vi "624WPI_DriverStationStart Communication.vi"(8 "error out":errorcluster, 11 "occurrence":refnum<k4>) -> ()   [LabVIEW 2013]
doc: "Starts the communication loop between the CompactRIO device and the driver station. This VI also initializes the host computer, joystick, and driver station data caches, as well as the system watchdog on the CompactRIO device.\n\nThis software is licensed. Open the labview\\readme\\WPI Robotics Library Open Source License.txt file for more information."
uses:
  <vilib>/Rock Robotics/WPI/DriverStation/WPI_DriverStationStatusErrorCache.ctl
  <vilib>/Rock Robotics/SystemInterfaces/NetworkCommunication/NetComm_UsageReport_ResourceType.ctl
  <vilib>/Rock Robotics/WPI/DriverStation/WPI_DriverStationLaptopDataCacheOp.ctl
  <vilib>/Rock Robotics/WPI/Joystick/WPI_JoystickCacheOp.ctl
  <vilib>/Rock Robotics/WPI/DriverStation/WPI_DriverStationCommDataCacheOp.ctl
  <vilib>/Rock Robotics/WPI/DriverStation/Enhanced IO/WPI_Enhanced IORaw Output Operation Mode.ctl
  <vilib>/Rock Robotics/WPI/DriverStation/WPI_DriverStationStatusDataCache.ctl
  <vilib>/Rock Robotics/WPI/Joystick/WPI_JoystickDeviceDataRaw.ctl
  <vilib>/Rock Robotics/WPI/DriverStation/WPI_DriverStationAllianceInfoCacheOp.ctl
  <vilib>/Rock Robotics/WPI/AnalogModule/WPI_AnalogModuleGetAverageVoltage.vi
  <vilib>/Utility/error.llb/Clear Errors.vi
panel:
  out "STOPCOMM":bool
  # "This VI start the communication loop and cache data for LabVIEW."
  # "VI MODIFIED - To use analog 8 (battery voltage) for speedier measurement\nin robot code, for correcting pressure readouts, etc."
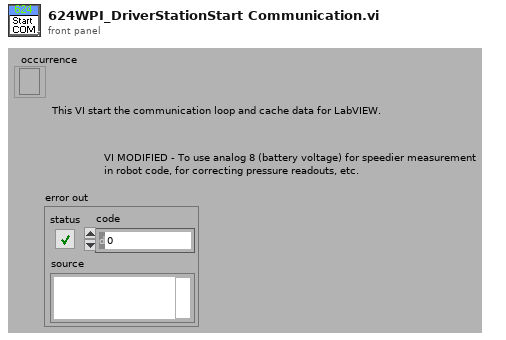
[diagram p1: front panel]
types:
  T1 = typedef "NetComm_UsageReport_ResourceType.ctl" = enum8{"Controller", "Module", "Language", "CANPlugin", "Accelerometer", "ADXL345", "AnalogChannel", "AnalogTrigger", "AnalogTriggerOutput", "CANJaguar", "Compressor", "Counter", "Dashboard", "DigitalInput", "DigitalOutput", "DriverStationCIO", "DriverStationEIO", "DriverStationLCD", "Encoder", "GearTooth", "Gyro", "I2C", "Framework", "Jaguar", "Joystick", "Kinect", "KinectStick", "PIDController", "Preferences", "PWM", "Relay", "RobotDrive", "SerialPort", "Servo", "Solenoid", "SPI", "Task", "Ultrasonic", "Victor", "Button", "Command", "AxisCamera", "PCVideoServer", "SmartDashboard", "Talon", "HiTechnicColorSensor", "HiTechnicAccel", "HiTechnicCompass", "SRF08"}
  T2 = typedef "WPI_DriverStationStatusErrorCache.ctl" = enum16{"Get", "Set"}
  T3 = typedef "WPI_DriverStationCommDataCacheOp.ctl" = enum16{"Get", "Set", "Init"}
  T4 = typedef "WPI_JoystickCacheOp.ctl" = enum16{"Set", "Init", "Get"}
  T5 = typedef "WPI_DriverStationLaptopDataCacheOp.ctl" = enum16{"Get", "Set", "Init"}
  T6 = typedef "WPI_JoystickDeviceDataRaw.ctl" = cluster{"axis 1":i8, "axis 2":i8, "axis 3":i8, "axis 4":i8, "axis 5":i8, "axis 6":i8, "Buttons":u16}
  T7 = typedef "WPI_DriverStationStatusDataCache.ctl" = enum16{"Get", "Set Digital Output", "Set High Priority Data", "Set Low Priority Data"}
  T8 = typedef "WPI_Enhanced IORaw Output Operation Mode.ctl" = enum16{"Get", "Set LEDs", "Set Digital Outputs", "Set Analog Outputs", "Set Digital Configuration", "Set PWMs", "Set All", "Invalidate", "Send Extended Bit", "Clear Extended Bit"}
  T9 = typedef "WPI_DriverStationAllianceInfoCacheOp.ctl" = enum16{"Get", "Set", "Init"}
  T10 = typedef "WPI_Enhanced IODataIn.ctl" = cluster{"api_version":u8, "fw_version":u8, "analog":cluster{"analog[0]":i16, "analog[1]":i16, "analog[2]":i16, "analog[3]":i16, "analog[4]":i16, "analog[5]":i16, "analog[6]":i16, "analog[7]":i16}, "digital":u16, "accel":cluster{"accel[0]":i16, "accel[1]":i16, "accel[2]":i16}, "quad":cluster{"quad[0]":i16, "quad[1]":i16}, "buttons":u8, "capsense slider":u8, "capsense prox":u8}
  T11 = typedef "WPI_Enhanced IODataOut.ctl" = cluster{"digital":u16, "digital_oe":u16, "digital_pe":u16, "pwm1_compare1":u16, "pwm1_compare2":u16, "pwm2_compare1":u16, "pwm2_compare2":u16, "pwm1_period":u16, "pwm2_period":u16, "dac1":u8, "dac2":u8, "leds":u8, "enables":u8, "dig_out":u8}
  T12 = typedef "WPI_DriverStationCommPacketData.ctl" = cluster{"packetIndex":u16, "control":u8, "dsDigitalIn":u8, "teamID":u16, "dsIDAlliance":u8, "dsIDPosition":u8, "J0 Axis 1":i8, "J0 Axis 2":i8, "J0 Axis 3":i8, "J0 Axis 4":i8, "J0 Axis 5":i8, "J0 Axis 6":i8, "J0 Buttons":u16, "J1 Axis 1":i8, "J1 Axis 2":i8, "J1 Axis 3":i8, "J1 Axis 4":i8, "J1 Axis 5":i8, "J1 Axis 6":i8, "J1 Buttons":u16, "J2 Axis 1":i8, "J2 Axis 2":i8, "J2 Axis 3":i8, "J2 Axis 4":i8, "J2 Axis 5":i8, "J2 Axis 6":i8, "J2 Buttons":u16, "J3 Axis 1":i8, "J3 Axis 2":i8, "J3 Axis 3":i8, "J3 Axis 4":i8, "J3 Axis 5":i8, "J3 Axis 6":i8, "J3 Buttons":u16, "analog 1":u16, "analog 2":u16, "analog 3":u16, "analog 4":u16, "cRIO checksum":u64, "FPGA checksum1":u64, "FPGA checksum2":u64, "vMonth1":u8, "vMonth2":u8, "vDay1":u8, "vDay2":u8, "vYear1":u8, "vYear2":u8, "vRev1":u8, "vRev2":u8}
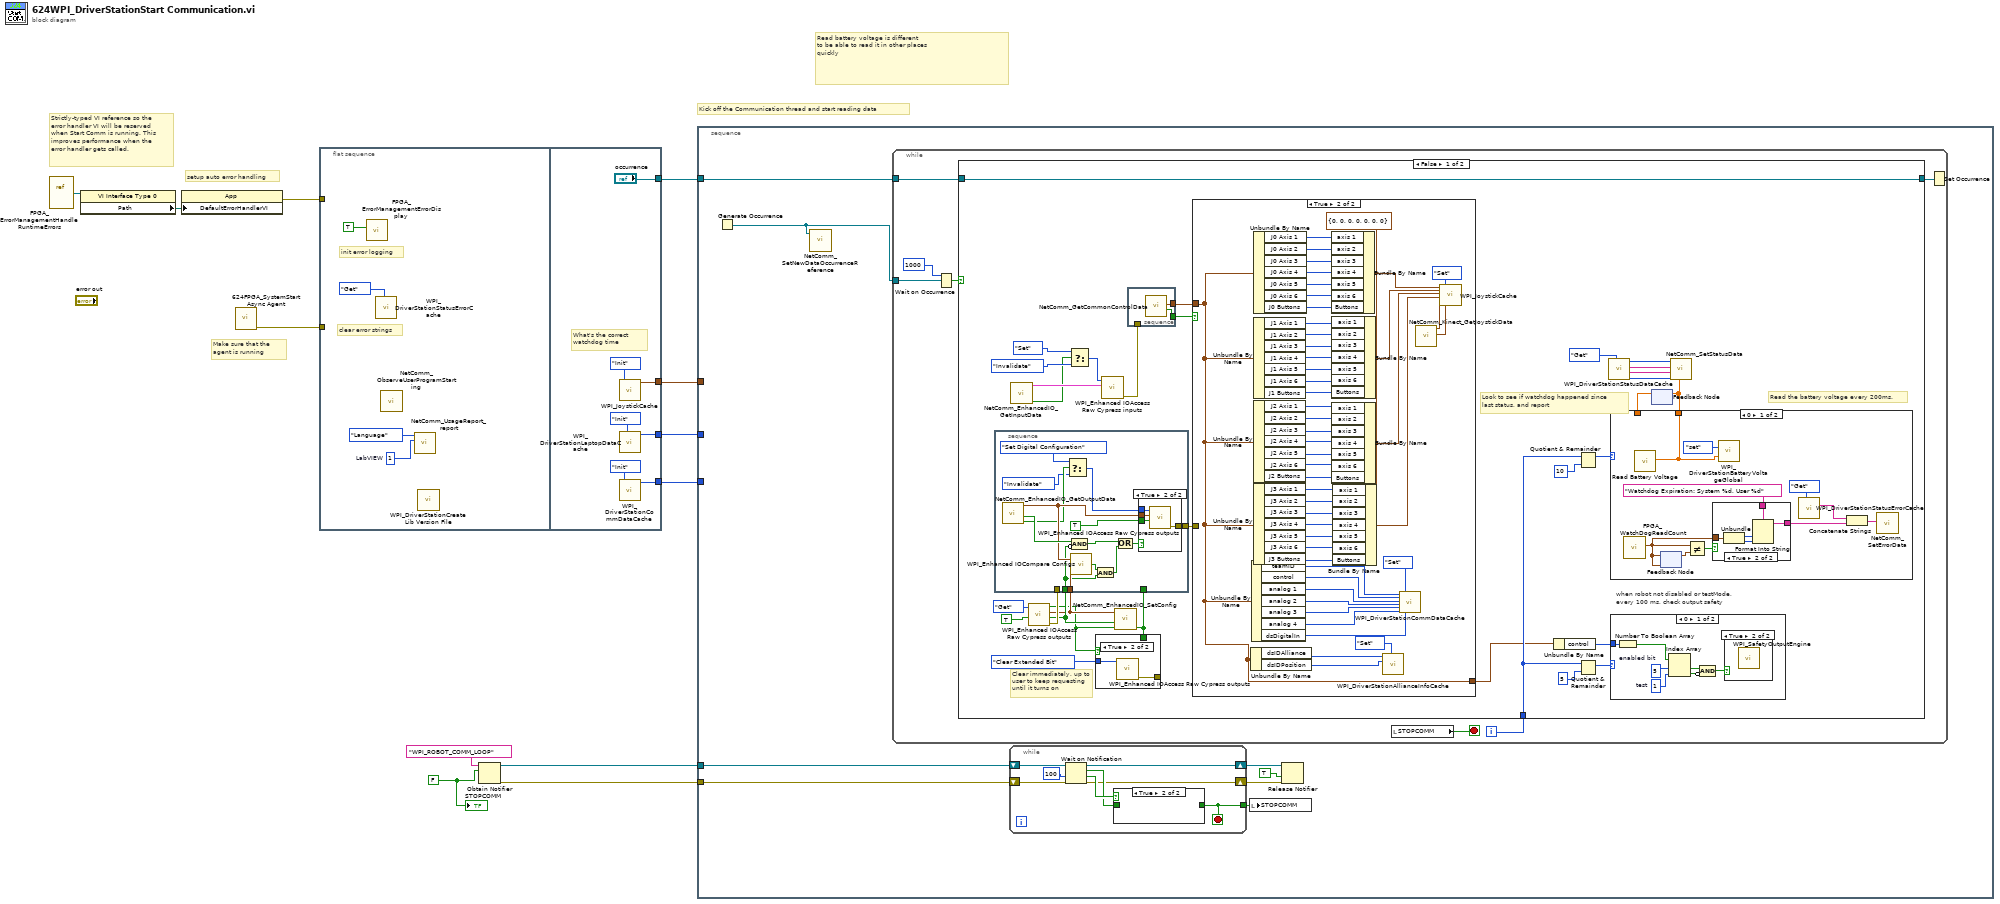
[diagram p0: block diagram]
diagram:
  w7 = FALSE
  # "setup auto error handling"
  # "Read battery voltage is different\nto be able to read it in other places\nquickly"
  # "Make sure that the\nagent is running"
  # "Strictly-typed VI reference so the error handler VI will be reserved when Start Comm is running. This improves performance when the error handler gets called."
  # "Kick off the Communication thread and start reading data"
  n1 = vi-ref <vilib>:"FPGA_ErrorManagementHandleRuntimeErrors.vi"() -> (w3:refnum<vi>)
  n2 = property class="VI Interface Type 0"(reference=w3) -> ("Path"=w2:path)  [unwired: 1 in, 2 out]
  n3 = property class="App"("DefaultErrorHandlerVI"=w2) -> (error out=w4:errorcluster)  [unwired: 2 in, 1 out]
  n4 = call "624FPGA_SystemStart Async Agent.vi"() -> ("error out"=w1:errorcluster)  [unwired: 11 in]
  n5 = flat-sequence {
    tunnel: w4 -> [_]
    tunnel: w1 -> [_]
    tunnel: [w23] -> w12
    tunnel: [w20] -> w11
    tunnel: [w18] -> w10
    tunnel: ["occurrence"] -> w5
    frame #0 {
      w14 = u8 1  # LabVIEW
      # "clear error strings"
      # "init error logging"
      n6 = call <vilib>:"FPGA_ErrorManagementErrorDisplay.vi"("Log to File (F)"=TRUE ("Log to File")) -> ()  [unwired: 2 in, 9 out]
      n7 = call <vilib>:"WPI_DriverStationStatusErrorCache.vi"("StatusErrorCacheOp"=WPI_DriverStationStatusErrorCache."Get") -> ()  [unwired: 1 in, 10 out]
      n8 = call <vilib>:"NetComm_ObserveUserProgramStarting.vi"() -> ()  [unwired: 1 out]
      n9 = call <vilib>:"NetComm_UsageReport_report.vi"("Instance Number"=w14, "Resource Type"=NetComm_UsageReport_ResourceType."Language") -> ()  [unwired: 10 in]
      n10 = call <vilib>:"WPI_DriverStationCreate Lib Version File.vi"() -> ()  [unwired: 12 in]
    }
    frame #1 {
      # "What's the correct watchdog time"
      n11 = call <vilib>:"WPI_JoystickCache.vi"("JoystickCacheOp"=WPI_JoystickCacheOp."Init") -> ("JoystickOut"=w20:T6)  [unwired: 7 in, 11 out]
      n12 = call <vilib>:"WPI_DriverStationLaptopDataCache.vi"("LaptopCacheOp"=WPI_DriverStationLaptopDataCacheOp."Init") -> ("Laptop Data Out"=w23:u8[])  [unwired: 10 out]
      n13 = call <vilib>:"WPI_DriverStationCommDataCache.vi"("CommDataCacheOp"=WPI_DriverStationCommDataCacheOp."Init") -> ("TeamID out"=w18:u16)  [unwired: 18 out]
    }
  }
  n14 = Obtain Notifier(name (unnamed)="WPI_ROBOT_COMM_LOOP", notification data type=w7) -> (notifier out=w8:refnum<notifier>, error out=w6:errorcluster)  [unwired: 2 in, 1 out]
  n15 = stacked-sequence {
    tunnel: w12 -> [_]
    tunnel: w11 -> [_]
    tunnel: w10 -> [_]
    tunnel: w8 -> [w31]
    tunnel: w6 -> [w27]
    tunnel: w5 -> [w24]
    frame #0 {
      n16 = Generate Occurrence() -> (w25:refnum<k4>)
      n17 = call <vilib>:"NetComm_SetNewDataOccurrenceReference.vi"("occurrence"=w25) -> ()  [unwired: 11 out]
      n18 = while {
        tunnel: w25 -> [w45]
        tunnel: w24 -> [w43]
        i -> [w41]
        stop <- w47 stop-if-true
        n19 = Wait on Occurrence(2:w45, 3:1000 ("ms timeout (-1)")) -> (0:w44:bool)  [unwired: 1 out]
        n20 = case shown="False" w44 {
          tunnel: w43 -> [w79 _]
          tunnel: [w79 _] -> w42
          tunnel: w41 -> [w72 _]
          frame False {
            # "Look to see if watchdog happened since\nlast status, and report"
            # "Read the battery voltage every 200ms."
            # "when robot not disabled or testMode,\nevery 100 ms, check output safety"
            # "Clear immediately, up to user to keep requesting until it turns on"
            n21 = call <vilib>:"NetComm_EnhancedIO_GetInputData.vi"() -> ("Success"=w58:bool, "Raw Data in"=w62:T10)  [unwired: 10 out]
            n22 = call <vilib>:"WPI_Enhanced IOAccess Raw Cypress outputs.vi"("Not API Call"=TRUE, "Data Operation"=WPI_Enhanced_IORaw_Output_Operation_Mode."Get") -> ("error out"=w77:errorcluster, "Config Affected"=w76:bool, "Raw Data Out"=w75:T11, "Extended Bit"=w68:bool)  [unwired: 2 in, 4 out]
            n23 = Select(t=enum16{"Get", "Set", "Invalidate"}."Set" ("Data Operation"), s=w58, f=enum16{"Get", "Set", "Invalidate"}."Invalidate" ("Data Operation")) -> (s? t:f=w61:enum16{"Get", "Set", "Invalidate"})
            n24 = call <vilib>:"WPI_Enhanced IOAccess Raw Cypress inputs.vi"("Raw Data in"=w62, "Data Operation"=w61) -> ("error out"=w57:errorcluster)  [unwired: 1 in, 8 out]
            n25 = call <vilib>:"NetComm_EnhancedIO_SetConfig.vi"("Send Extended Bit"=w68, "Config Changed"=w76, "DataOut"=w75) -> ("Success"=w65:bool)  [unwired: 8 out]
            n26 = stacked-sequence {
              tunnel: w65 -> [_]
              tunnel: w77 -> [_]
              tunnel: w76 -> [w113]
              tunnel: w75 -> [w115]
              tunnel: [w107] -> w63
              frame #0 {
                n27 = call <vilib>:"NetComm_EnhancedIO_GetOutputData.vi"() -> ("Success"=w110:bool, "Config Chg"=w118:bool, "DataOut"=w116:T11)  [unwired: 9 out]
                n28 = Select(t=WPI_Enhanced_IORaw_Output_Operation_Mode."Set Digital Configuration" ("Data Operation"), s=w110, f=WPI_Enhanced_IORaw_Output_Operation_Mode."Invalidate" ("Data Operation")) -> (s? t:f=w120:T8)
                n29 = call <vilib>:"WPI_Enhanced IOCompare Configs.vi"("Raw Data Out"=w115, "DataOut"=w116) -> ("Config Equal"=w114:bool)
                n30 = Compound Arithmetic op=AND(w118, invert w113) -> (w117:bool)
                n31 = Compound Arithmetic op=AND(w114, w113) -> (w111:bool)
                n32 = Or(x=w117, y=w111) -> (x .or. y?=w112:bool)
                n33 = case shown="True" w112 {
                  tunnel: w116 -> [_ w124]
                  tunnel: w120 -> [_ w123]
                  tunnel: TRUE ("Not API Call") -> [_ w122]
                  tunnel: [_ w121] -> w107
                  frame False {
                  }
                  frame True {
                    n34 = call <vilib>:"WPI_Enhanced IOAccess Raw Cypress outputs.vi"("Not API Call"=w122, "Raw Data In"=w124, "Data Operation"=w123) -> ("error out"=w121:errorcluster)  [unwired: 1 in, 7 out]
                  }
                }
              }
            }
            n35 = case shown="True" w68 {
              tunnel: WPI_Enhanced_IORaw_Output_Operation_Mode."Clear Extended Bit" ("Data Operation") -> [_ w99]
              tunnel: [_ w98] -> _
              tunnel: w65 -> [_ _]
              frame False {
              }
              frame True {
                n36 = call <vilib>:"WPI_Enhanced IOAccess Raw Cypress outputs.vi"("Data Operation"=w99) -> ("error out"=w98:errorcluster)  [unwired: 3 in, 7 out]
              }
            }
            n37 = stacked-sequence {
              tunnel: [w97] -> w64
              tunnel: [w96] -> w70
              tunnel: w57 -> [_]
              frame #0 {
                n38 = call <vilib>:"NetComm_GetCommonControlData.vi"() -> ("New Data"=w97:bool, "FRC Control Data"=w96:T12)  [unwired: 3 in, 7 out]
              }
            }
            n39 = case shown="True" w64 {
              tunnel: w70 -> [w125 w126]
              tunnel: [w125 w126] -> w67
              tunnel: w63 -> [_ _]
              frame False {
              }
              frame True {
                w134 = T6 {"axis 1"=0, "axis 2"=0, "axis 3"=0, "axis 4"=0, "axis 5"=0, "axis 6"=0, "Buttons"=0} ("Joystick")
                n40 = Unbundle By Name(w126) -> ("dsIDAlliance"=w130:u8, "dsIDPosition"=w129:u8)
                n41 = Unbundle By Name(w126) -> ("teamID"=w135:u16, "control"=w136:u8, "analog 1"=w140:u16, "analog 2"=w139:u16, "analog 3"=w138:u16, "analog 4"=w132:u16, "dsDigitalIn"=w137:u8)
                n42 = Unbundle By Name(w126) -> ("J1 Axis 1"=w161:i8, "J1 Axis 2"=w160:i8, "J1 Axis 3"=w159:i8, "J1 Axis 4"=w158:i8, "J1 Axis 5"=w157:i8, "J1 Axis 6"=w156:i8, "J1 Buttons"=w155:u16)
                n43 = Unbundle By Name(w126) -> ("J2 Axis 1"=w154:i8, "J2 Axis 2"=w153:i8, "J2 Axis 3"=w152:i8, "J2 Axis 4"=w151:i8, "J2 Axis 5"=w150:i8, "J2 Axis 6"=w149:i8, "J2 Buttons"=w148:u16)
                n44 = Unbundle By Name(w126) -> ("J3 Axis 1"=w147:i8, "J3 Axis 2"=w146:i8, "J3 Axis 3"=w145:i8, "J3 Axis 4"=w144:i8, "J3 Axis 5"=w143:i8, "J3 Axis 6"=w142:i8, "J3 Buttons"=w141:u16)
                n45 = Unbundle By Name(w126) -> ("J0 Axis 1"=w168:i8, "J0 Axis 2"=w167:i8, "J0 Axis 3"=w166:i8, "J0 Axis 4"=w165:i8, "J0 Axis 5"=w164:i8, "J0 Axis 6"=w163:i8, "J0 Buttons"=w162:u16)
                n46 = Bundle By Name(cluster=w134, "axis 1"=w168, "axis 2"=w167, "axis 3"=w166, "axis 4"=w165, "axis 5"=w164, "axis 6"=w163, "Buttons"=w162) -> (w171:T6)
                n47 = Bundle By Name(cluster=w134, "axis 1"=w161, "axis 2"=w160, "axis 3"=w159, "axis 4"=w158, "axis 5"=w157, "axis 6"=w156, "Buttons"=w155) -> (w170:T6)
                n48 = Bundle By Name(cluster=w134, "axis 1"=w154, "axis 2"=w153, "axis 3"=w152, "axis 4"=w151, "axis 5"=w150, "axis 6"=w149, "Buttons"=w148) -> (w133:T6)
                n49 = Bundle By Name(cluster=w134, "axis 1"=w147, "axis 2"=w146, "axis 3"=w145, "axis 4"=w144, "axis 5"=w143, "axis 6"=w142, "Buttons"=w141) -> (w169:T6)
                n50 = call <vilib>:"WPI_DriverStationAllianceInfoCache.vi"("AllianceInfoCacheOp"=WPI_DriverStationAllianceInfoCacheOp."Set", "dsIDPosition"=w129, "dsIDAlliance"=w130) -> ()  [unwired: 9 out]
                n51 = call <vilib>:"WPI_DriverStationCommDataCache.vi"("TeamID"=w135, "ControlBit"=w136, "Analog1"=w140, "Analog2"=w139, "Analog3"=w138, "Analog4"=w132, "CommDataCacheOp"=WPI_DriverStationCommDataCacheOp."Set", "Digital"=w137) -> ()  [unwired: 12 out]
                n52 = call <vilib>:"NetComm_Kinect_GetJoystickData.vi"() -> ("Raw Joystick 2"=w127:T6, "Raw Joystick"=w128:T6)  [unwired: 9 in, 1 out]
                n53 = call <vilib>:"WPI_JoystickCache.vi"("Joystick"=w171, "Joystick 1"=w170, "Joystick 2"=w133, "Joystick 3"=w169, "Joystick 4"=w128, "JoystickCacheOp"=WPI_JoystickCacheOp."Set", "Joystick 5"=w127) -> ()  [unwired: 1 in, 12 out]
              }
            }
            n54 = Unbundle By Name(w67) -> ("control"=w66:u8)
            n55 = Quotient & Remainder(x=w72, y=u32 10 ("milliseconds to wait")) -> (x-y*floor(x/y)=w55:u32)  [unwired: 1 out]
            n56 = Quotient & Remainder(x=w72, y=u32 5 ("milliseconds to wait")) -> (x-y*floor(x/y)=w73:u32)  [unwired: 1 out]
            n57 = call <vilib>:"WPI_DriverStationStatusDataCache.vi"("StatusDataCacheOp"=WPI_DriverStationStatusDataCache."Get") -> ("Update Number"=w50:u8, "Low Priority Out"=w51:string, "High Priority Out"=w52:string, "Digital Output Out"=w53:u8)  [unwired: 3 in, 4 out]
            n58 = case shown="0" w73 {
              tunnel: w66 -> [w106 _]
              frame 0 {
                w103 = 1  # test
                w105 = 5  # enabled bit
                n59 = Number To Boolean Array(number=w106) -> (Boolean array=w104:bool[])
                n60 = Index Array(array=w104, index #1=w105, index #2=w103) -> (element #1=w100:bool, element #2=w101:bool)
                n61 = Compound Arithmetic op=AND(w100, invert w101) -> (w102:bool)
                n62 = case shown="True" w102 {
                  frame False {
                  }
                  frame True {
                    n63 = call <vilib>:"WPI_SafetyOutputEngine.vi"() -> ()  [unwired: 1 out]
                  }
                }
              }
              frame Default {
              }
            }
            n64 = feedback #1() -> (w54:dbl)  [unwired: 1 out]
            n65 = case shown="0" w55 {
              tunnel: w54 -> [_ w95]
              tunnel: [w80 w95] -> w49
              frame 0 {
                n66 = call <vilib>:"FPGA_WatchDogReadCount.vi"() -> ("Counts"=w85:cluster{"System":i32, "User":i32})  [unwired: 1 in, 10 out]
                n67 = call "Read Battery Voltage.vi"() -> ("Voltage"=w80:dbl)  [unwired: 11 in]
                n68 = feedback #2(w85) -> (w83:cluster{"System":i32, "User":i32})
                n69 = feedback-in #2(w85) -> ()
                n70 = Not Equal?(x=w85, y=w83) -> (x != y?=w81:bool)
                n71 = case shown="True" w81 {
                  tunnel: w85 -> [_ w94]
                  tunnel: "Watchdog Expiration: System %d, User %d" ("Error Strings out") -> [_ w91]
                  tunnel: [_ w90] -> w82
                  frame False {
                  }
                  frame True {
                    n72 = Unbundle(w94) -> ("System"=w93:i32, "User"=w92:i32)
                    n73 = Format Into String(format string=w91, w93, w92) -> (resulting string=w90:string)  [unwired: 2 in, 1 out]
                  }
                }
                n74 = call <vilib>:"WPI_DriverStationBatteryVoltageGlobal.vi"("menu"=enum16{"set", "get"}."set", "battery voltage in"=w80) -> ()  [unwired: 13 in, 1 out]
                n75 = call <vilib>:"WPI_DriverStationStatusErrorCache.vi"("StatusErrorCacheOp"=WPI_DriverStationStatusErrorCache."Get") -> ("Error Strings out"=w87:string)  [unwired: 1 in, 9 out]
                n76 = Concatenate Strings(w87, w82) -> (w88:string)
                n77 = call <vilib>:"NetComm_SetErrorData.vi"("Error Data"=w88) -> ()  [unwired: 3 in, 8 out]
              }
              frame 1, Default {
              }
            }
            n78 = feedback-in #1(w49) -> ()
            n79 = call <vilib>:"NetComm_SetStatusData.vi"("Battery"=w49, "Update Number"=w50, "Low Priority User Data"=w51, "High Priority User Data"=w52, "Digital Output"=w53) -> ()  [unwired: 1 in, 6 out]
          }
          frame True {
          }
        }
        n80 = local read "STOPCOMM"() -> (w47:bool)
        n81 = Set Occurrence(w42) -> ()
      }
      n82 = while {
        shift-right: [w35] -> w29
        shift-left: w31 -> [w38]
        tunnel: [w34] -> w30
        shift-right: [w33] -> w26
        shift-left: w27 -> [w32]
        stop <- w34 stop-if-true
        n83 = Wait on Notification(notifier=w38, timeout in ms (-1)=100, error in (no error)=w32) -> (notifier out=w35:refnum<notifier>, notification=w36:bool, timed out?=w37:bool, error out=w33:errorcluster)  [unwired: 1 out]
        n84 = case shown="True" w37 {
          tunnel: w36 -> [w40 _]
          tunnel: [w40 _] -> w34
          frame False {
          }
          frame True {
          }
        }
      }
      n85 = local write "STOPCOMM"(w30) -> ()
      n86 = Release Notifier(notifier=w29, force destroy? (F)=TRUE, error in (no error)=w26) -> ()  [unwired: 3 out]
    }
  }
  "STOPCOMM" <- w7
